vi "Write Single padded pulse.vi"(8 "error in (no error)":errorcluster, 10 "Single padded pulse":i8[](array[numeric]), 11 "Combine_pulses in":refnum<class "Combine_pulses.lvclass">) -> (0 "error out":errorcluster, 3 "Combine_pulses out":refnum<class "Combine_pulses.lvclass">)   [LabVIEW 2019, in "Combine_pulses.lvclass"]
uses:
  Combine_pulses.lvclass
  Combine_pulses.lvclass/Combine_pulses.ctl
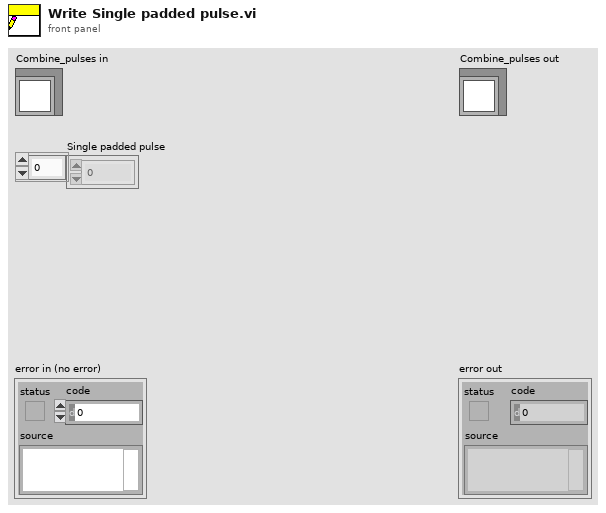
[diagram p1: front panel]
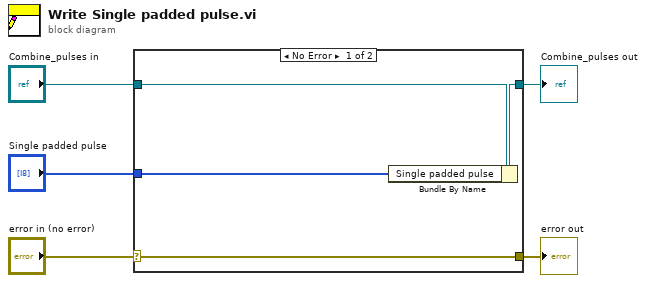
[diagram p0: block diagram]
diagram:
  n1 = case shown="No Error" "error in (no error)" {
    selector: "error in (no error)" -> [w9 w10]
    tunnel: [w9 w10] -> w4
    tunnel: [w7 w11] -> w2
    tunnel: "Combine_pulses in" -> [w8 w11]
    tunnel: "Single padded pulse" -> [w6 _]
    frame No Error {
      n2 = Bundle By Name(cluster=w8, "Single padded pulse"=w6) -> (w7:refnum<class "Combine_pulses.lvclass">)
    }
    frame Error {
    }
  }
  "error out" <- w4
  "Combine_pulses out" <- w2
